vi "PV HLT5xx Miscellaneous.vi"(8 "error in (no error)":errorcluster, 9 "PV Miscellaneous - Cluster":T1={"Parameter"=0, "Parameter\nread only<->describe"=FALSE, "Unit adress"=1, "Altn Protocol"=0} {"Altn Protocol" items=["PV Protocol", "HLT5xx-Protocol", "Inficon Binär"]; "Unit adress" min=1 max=255 step=1; "Parameter" items=[" Actual error code (read only)", " Alternative Protocol", " Unit adress", " Error acknowledgement (write only)"]}, 10 "Adress of unit":u16=1 max=999 step=1, 11 "VISA session":refnum<visa-resource-name>) -> (0 "error out":errorcluster, 2 "response (data)":string, 3 "dup VISA session":refnum<visa-resource-name>)   [LabVIEW 2021, in "Pfeiffer Vacuum.lvlib"]
doc: "There are 4 parameters available, only one of which can be enabled at a time. \n\n0 - Actual error code (read only) (default) - Para 303\n1 - Alternative Protocol - Para 089\n2 - Unit adress - Para797\n3 - Error acknowledgement (write only) - Para 009\n\nNote: The 2 controls right of this one will set the appropriate values for the selected parameter. Any settings for an parameter that is not selected will be ignored. If a value is out of range, it will be changed to either the upper or the lower limit of the range."
uses:
  <instrlib>/Pfeiffer Vacuum/Pfeiffer Vacuum.lvlib
  <instrlib>/Pfeiffer Vacuum/Public/LeakDetector/PV HLT5xx Miscellaneous - Cluster.ctl
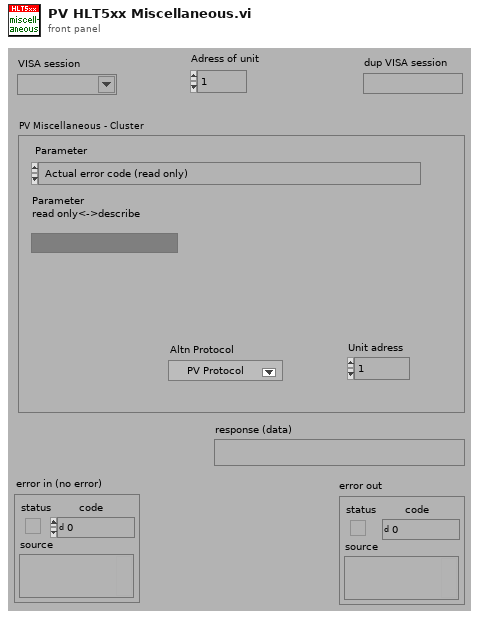
[diagram p1: front panel]
types:
  T1 = typedef "PV HLT5xx Miscellaneous - Cluster.ctl" = cluster{"Parameter":u16, "Parameter\nread only<->describe":bool, "Unit adress":i16, "Altn Protocol":u16}
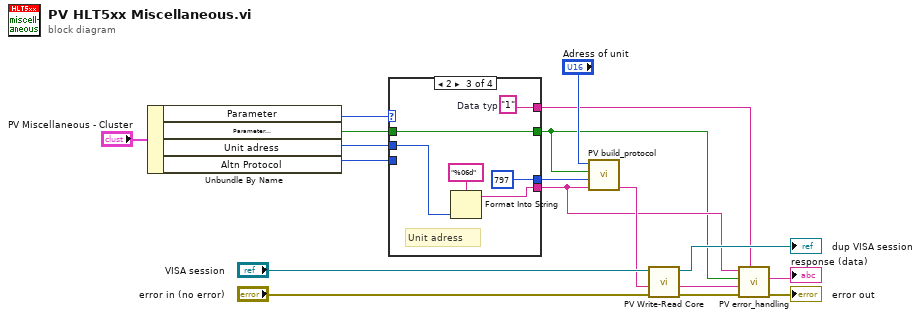
[diagram p0: block diagram]
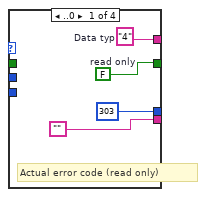
[diagram p2: hidden frame]
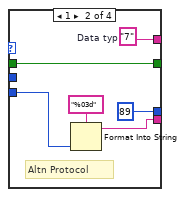
[diagram p3: hidden frame]
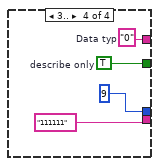
[diagram p4: hidden frame]
diagram:
  n1 = Unbundle By Name("PV Miscellaneous - Cluster") -> ("Parameter"=w15:u16, "Parameter\nread only<->describe"=w14:bool, "Unit adress"=w12:i16, "Altn Protocol"=w1:u16)
  n2 = case shown="2" w15 {
    tunnel: [u16 303 ("Parameter-number") u16 89 ("Parameter-number") u16 797 ("Parameter-number") u16 9 ("Parameter-number")] -> w17
    tunnel: ["" w27 w33 "111111" ("Data")] -> w4
    tunnel: [w21 w25 w31 w38] -> w3
    tunnel: w14 -> [_ w25 w31 _]
    tunnel: w12 -> [_ _ w30 _]
    tunnel: [w19 w24 w29 w35] -> w5
    tunnel: w1 -> [_ w23 _ _]
    frame ..0 {
      w19 = "4"  # Data typ
      w21 = FALSE  # read only
      # "Actual error code (read only)"
    }
    frame 1 {
      w24 = "7"  # Data typ
      # "Altn Protocol"
      n3 = Format Into String(format string="%03d" ("Format-String"), w23) -> (resulting string=w27:string)  [unwired: 2 in, 1 out]
    }
    frame 2 {
      w29 = "1"  # Data typ
      # "Unit adress"
      n4 = Format Into String(format string="%06d" ("Format-String"), w30) -> (resulting string=w33:string)  [unwired: 2 in, 1 out]
    }
    frame 3.. {
      w35 = "0"  # Data typ
      w38 = TRUE  # describe only
    }
  }
  n5 = call <instrlib>:"PV build_protocol.vi"("Data"=w4, "Parameter-number"=w17, "parameter\nread<->describe"=w3, "Adress"="Adress of unit") -> ("output"=w9:string)  [unwired: 3 in]
  n6 = call <instrlib>:"PV Write-Read Core.vi"("error in"="error in (no error)", "Write data in"=w9, "VISA session"="VISA session") -> ("error out"=w6:errorcluster, "response (data) out"=w7:string, "dup VISA session"=→"dup VISA session":refnum<visa-resource-name>)  [unwired: 2 in]
  n7 = call <instrlib>:"PV error_handling.vi"("Data Typ in"=w5, "error in"=w6, "response (data) in"=w7, "Parameter\nread only<->describe"=w3, "data in"=w4) -> ("error out"=→"error out":errorcluster, "Data out"=→"response (data)":string)  [unwired: 4 in, 1 out]
